vi "String to Array.vi"(1 "String":string) -> (0 "Array":u16[](array[numeric]))   [LabVIEW 2015]
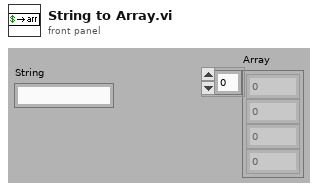
[diagram p1: front panel]
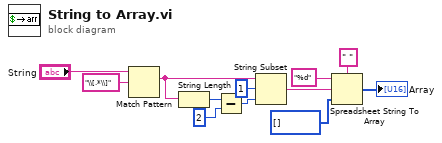
[diagram p0: block diagram]
diagram:
  n1 = Match Pattern(string="String", regular expression="\\[.*\\]") -> (match substring=w9:string)  [unwired: 1 in, 3 out]
  n2 = String Length(string=w9) -> (length=w8:i32)
  n3 = Subtract(x=w8, y=2) -> (x-y=w6:i32)
  n4 = String Subset(string=w9, offset (0)=1, length (rest)=w6) -> (substring=w1:string)
  n5 = Spreadsheet String To Array(delimiter (Tab)=" ", format string="%d" ("spreadsheet string"), spreadsheet string=w1, array type (2D Dbl)=u16[] [] ("Array")) -> (array=→"Array":u16[])
